vi "Hash File with SHA-256.vi"(8 "error In":errorcluster, 11 "Path to Hash":path) -> (0 "error Out":errorcluster, 3 "Hash String":string)   [LabVIEW 2012, in "SHA256.lvlib"]
doc: "Calculates the SHA-256 hash for a file on dosc."
uses:
  SHA256.lvlib
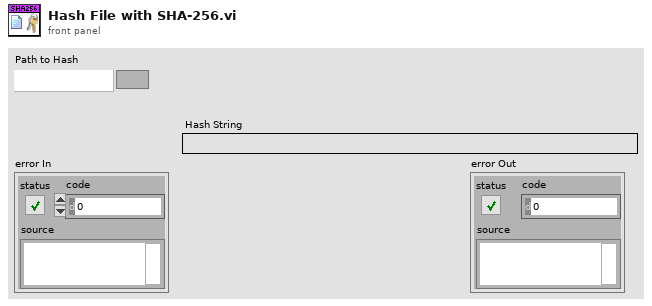
[diagram p1: front panel]
types:
  T1 = enum16{"big-endian, network order", "native, host order", "little-endian"}
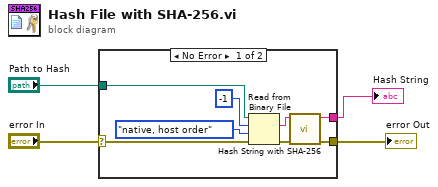
[diagram p0: block diagram]
diagram:
  n1 = case shown="No Error" "error In" {
    selector: "error In" -> [w9 w13]
    tunnel: "Path to Hash" -> [w12 _]
    tunnel: [w6 w13] -> w2
    tunnel: [w5 _] -> w1
    frame No Error {
      n2 = Read from Binary File(8:w9, 9:T1."native, host order" ("byte order (0:big-endian, network order)"), 10:-1 ("count (1)"), 11:w12) -> (0:w7:errorcluster, 2:w8:string)  [unwired: 2 in, 2 out]
      n3 = call "Hash String with SHA-256.vi"("error In"=w7, "String to Encode"=w8) -> ("error Out"=w6:errorcluster, "Hash String"=w5:string)  [unwired: 8 in]
    }
    frame Error {
    }
  }
  "Hash String" <- w1
  "error Out" <- w2
